vi "v2.0.vi"() -> ()   [LabVIEW 2018]
uses:
  <vilib>/DAQmx/read.llb/DAQmx Read (Analog 1D DBL NChan 1Samp).vi
  <vilib>/DAQmx/create/channels.llb/DAQmx Create Channel (AI-Voltage-Basic).vi
  <vilib>/DAQmx/configure/timing.llb/DAQmx Timing (Sample Clock).vi
  <vilib>/DAQmx/miscellaneous.llb/DAQmx Fill In Error Info.vi
panel:
  out "Status":T1(ring)
  out "Live Display":dbl[](array[numeric])
  in  "Stop":bool
  in  "OK Button":bool
  in  "DAQ Properties":cluster{"Sample Rate":dbl}
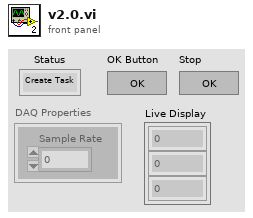
[diagram p1: front panel]
types:
  T1 = enum16{"Create Task", "Change Settings", "Check Settings", "Read Data", "End Task"}
  T2 = enum8{"Enabled", "Disabled", "Disabled and Grayed Out"}
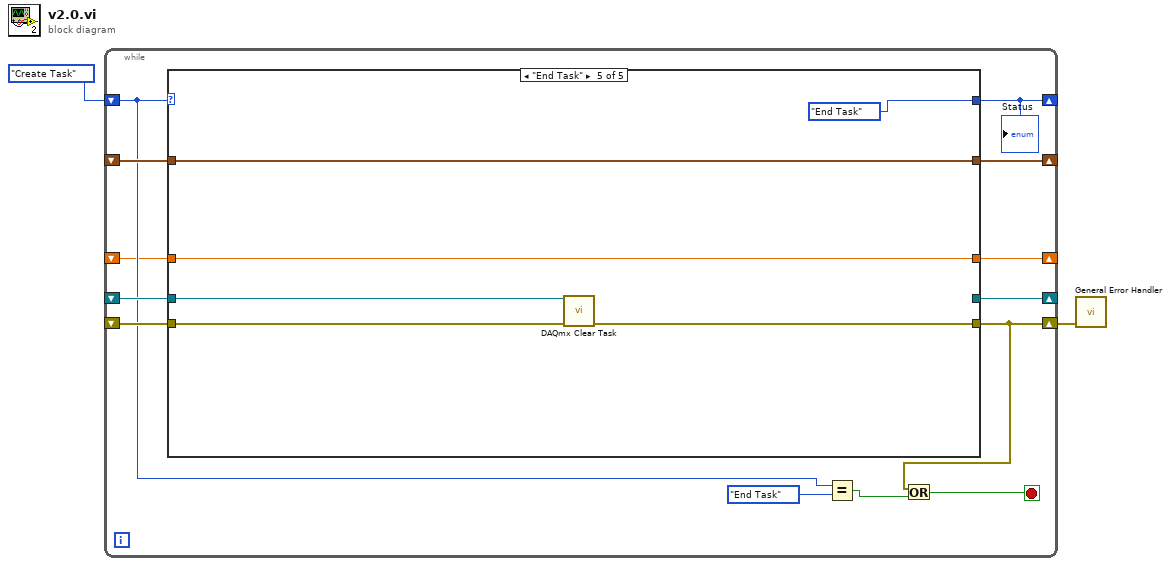
[diagram p0: block diagram]
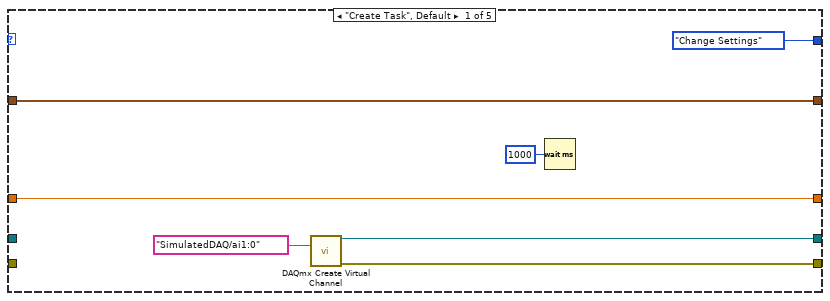
[diagram p2: hidden frame]
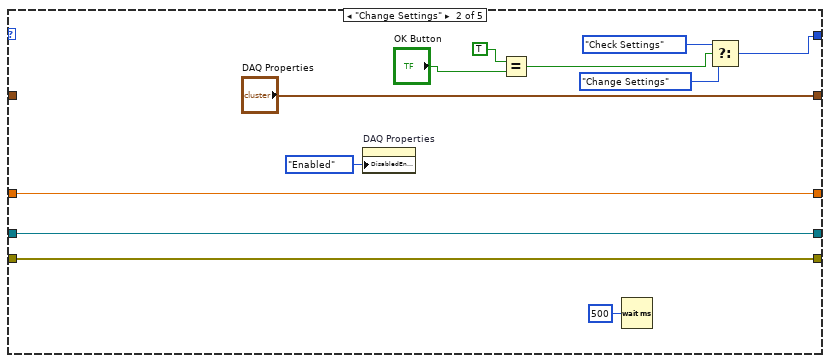
[diagram p3: hidden frame]
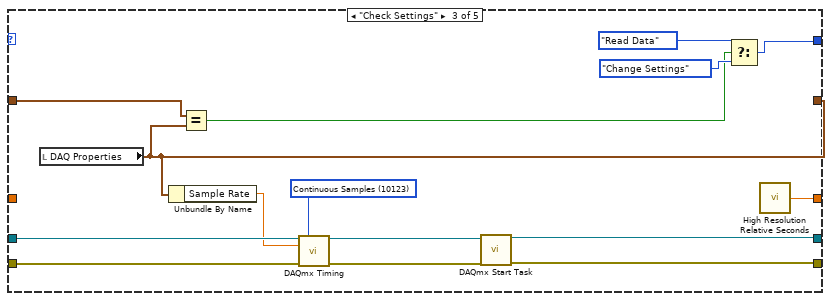
[diagram p4: hidden frame]
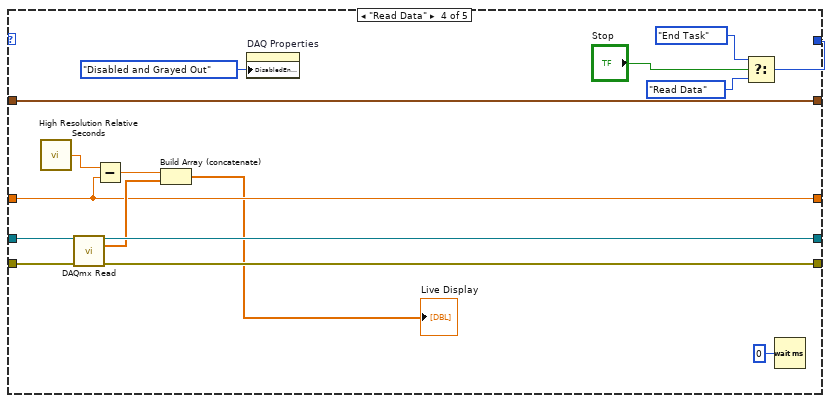
[diagram p5: hidden frame]
diagram:
  n1 = while {
    shift-right: [w10] -> _
    shift-left: T1."Create Task" -> [w5]
    shift-right: [w15] -> _
    shift-left: _ -> [w13]
    shift-right: [w9] -> w1
    shift-left: _ -> [w12]
    shift-right: [w14] -> _
    shift-left: _ -> [w11]
    shift-right: [w4] -> _
    shift-left: _ -> [w3]
    stop <- w8 stop-if-true
    n2 = case shown="\"End Task\"" w5 {
      tunnel: [w22 w34 w39 w62 _] -> w15
      tunnel: [w21 w33 w38 w61 w71] -> w9
      tunnel: [T1."Change Settings" w27 w46 w59 T1."End Task"] -> w10
      tunnel: [w18 "DAQ Properties" w42 w63 w70] -> w14
      tunnel: w13 -> [_ w34 w45 w65 w68]
      tunnel: w12 -> [_ w33 w44 w64 w67]
      tunnel: w11 -> [w18 _ w49 w63 w70]
      tunnel: [w16 w24 w35 w52 w66] -> w4
      tunnel: w3 -> [w16 w24 _ w52 w66]
      frame "Create Task", Default {
        n3 = call-poly <vilib>:"DAQmx Create Virtual Channel.vi"("physical channels"=tag "SimulatedDAQ/ai1:0") -> ("task out"=w22:refnum<k21>, "error out"=w21:errorcluster)  [unwired: 13 in]
        n4 = Wait (ms)(milliseconds to wait=u32 1000) -> ()  [unwired: 1 out]
      }
      frame "Change Settings" {
        n5 = property on="DAQ Properties" class="Clust (strict)"("DisabledEnum"=T2."Enabled" ("Disabled")) -> ()  [unwired: 2 in, 2 out]
        n6 = Equal?(x=TRUE, y="OK Button") -> (x = y?=w29:bool)
        n7 = Wait (ms)(milliseconds to wait=u32 500) -> ()  [unwired: 1 out]
        n8 = Select(t=T1."Check Settings", s=w29, f=T1."Change Settings") -> (s? t:f=w27:T1)
      }
      frame "Check Settings" {
        w36 = 10123 items=["Finite Samples"=10178, "Continuous Samples"=10123, "Hardware Timed Single Point"=12522] ("sample mode")
        n9 = local read "DAQ Properties"() -> (w42:cluster{"Sample Rate":dbl})
        n10 = Unbundle By Name(w42) -> ("Sample Rate"=w43:dbl)
        n11 = Equal?(x=w49, y=w42) -> (x = y?=w37:bool)
        n12 = call-poly <vilib>:"DAQmx Timing.vi"("task/channels in"=w45, "sample mode"=w36, "rate"=w43, "error in"=w44) -> ("task out"=w41:refnum<k21>, "error out"=w40:errorcluster)  [unwired: 10 in]
        n13 = call <vilib>:"DAQmx Start Task.vi"("task/channels in"=w41, "error in"=w40) -> ("task out"=w39:refnum<k21>, "error out"=w38:errorcluster)  [unwired: 12 in]
        n14 = Select(t=T1."Read Data", s=w37, f=T1."Change Settings") -> (s? t:f=w46:T1)
        n15 = call <vilib>:"High Resolution Relative Seconds.vi"() -> ("relative seconds"=w35:dbl)
      }
      frame "Read Data" {
        n16 = call <vilib>:"High Resolution Relative Seconds.vi"() -> ("relative seconds"=w55:dbl)
        n17 = call-poly <vilib>:"DAQmx Read.vi"("task/channels in"=w65, "error in"=w64) -> ("task out"=w62:refnum<k21>, "data"=w54:dbl[], "error out"=w61:errorcluster)  [unwired: 11 in]
        n18 = Subtract(x=w55, y=w52) -> (x-y=w53:dbl)
        n19 = Build Array (concatenate)(w53, w54) -> (→"Live Display":dbl[])
        n20 = property on="DAQ Properties" class="Clust (strict)"("DisabledEnum"=T2."Disabled and Grayed Out" ("Disabled")) -> ()  [unwired: 2 in, 2 out]
        n21 = Select(t=T1."End Task", s="Stop", f=T1."Read Data") -> (s? t:f=w59:T1)
        n22 = Wait (ms)(milliseconds to wait=u32 0) -> ()  [unwired: 1 out]
      }
      frame "End Task" {
        n23 = call <vilib>:"DAQmx Clear Task.vi"("task in"=w68, "error in"=w67) -> ("error out"=w71:errorcluster)  [unwired: 13 in]
      }
    }
    "Status" <- w10
    n24 = Equal?(x=w5, y=T1."End Task") -> (x = y?=w6:bool)
    n25 = Or(x=w9, y=w6) -> (x .or. y?=w8:bool)
  }
  n26 = call <vilib>:"General Error Handler.vi"("error in (no error)"=w1) -> ()  [unwired: 10 in, 5 out]
